vi "st_Geometric CDF (kx).vi"(10 "p":dbl=0.5, 11 "nx":dbl=1.0) -> (0 "error":i32, 3 "cdf(nx)":dbl=0.75)   [LabVIEW 2020, in "NI_Gmath.lvlib"]
uses:
  NI_Gmath.lvlib
  st_error_code.ctl
panel:
  # "Geometric CDF"
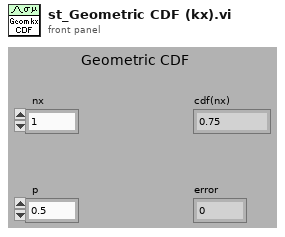
[diagram p1: front panel]
types:
  T1 = typedef "NI_Gmath.lvlib/st_error_code.ctl" = i32
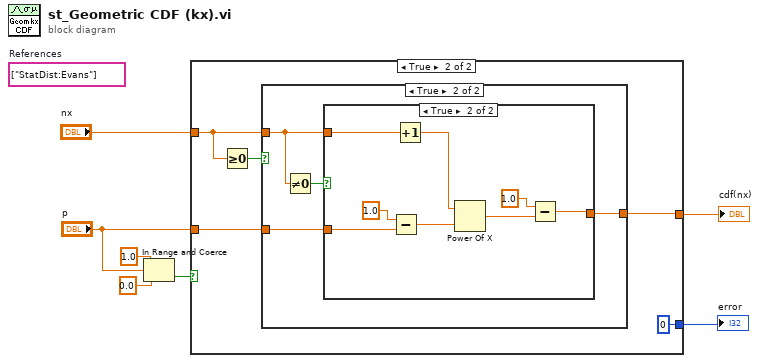
[diagram p0: block diagram]
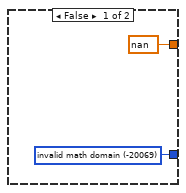
[diagram p2: hidden frame]
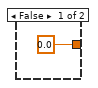
[diagram p3: hidden frame]
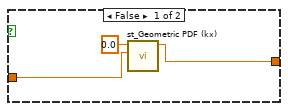
[diagram p4: hidden frame]
diagram:
  (unwired) string[] ["StatDist:Evans"]  # References
  n1 = In Range and Coerce(upper limit=1.0, x="p", lower limit=0.0) -> (In Range?=w4:bool)  [unwired: 1 out]
  n2 = case shown="True" w4 {
    tunnel: [w8 0 ("invalid math domain")] -> w7
    tunnel: [nan w12] -> w6
    tunnel: "nx" -> [_ w10]
    tunnel: "p" -> [_ w11]
    frame False {
      w8 = T1 -20069 items=["invalid math domain"=-20069, "Fourier interpolation size m >= n"=-20070, "empty array"=-20003] ("stat interp error code")
    }
    frame True {
      n3 = Greater Or Equal To 0?(x=w10) -> (x >= 0?=w13:bool)
      n4 = case shown="True" w13 {
        tunnel: [0.0 w19] -> w12
        tunnel: w11 -> [_ w18]
        tunnel: w10 -> [_ w17]
        frame False {
        }
        frame True {
          n5 = Not Equal To 0?(x=w17) -> (x != 0?=w16:bool)
          n6 = case shown="True" w16 {
            tunnel: w17 -> [_ w28]
            tunnel: [w20 w24] -> w19
            tunnel: w18 -> [w21 w27]
            frame False {
              n7 = call "st_Geometric PDF (kx).vi"("p"=w21, "x"=0.0) -> ("pdf(x)"=w20:dbl)  [unwired: 8 in, 1 out]
            }
            frame True {
              n8 = Subtract(x=1.0, y=w27) -> (x-y=w29:dbl)
              n9 = Increment(x=w28) -> (x+1=w26:dbl)
              n10 = Power Of X(1:w29, 2:w26) -> (0:w23:dbl)
              n11 = Subtract(x=1.0, y=w23) -> (x-y=w24:dbl)
            }
          }
        }
      }
    }
  }
  "cdf(nx)" <- w6
  "error" <- w7
